vi "pH电极校准.vi"() -> ()   [LabVIEW 2016, in "斯坦道多参数.lvlib"]
uses:
  <vilib>/Utility/miscctls.llb/LVPointTypeDef.ctl
  <vilib>/Analysis/NI_AALBase.lvlib
panel:
  out "滤波设定":dbl
  in  "刷新按钮":bool
  out "第三点信号值":dbl
  out "第二点信号值":dbl
  out "第一点信号值":dbl
  out "温度":dbl format="%#.2f"
  out "通讯状态":string
  out "电极状态标志":u16(ring) items=["OK", "第一点校正通过", "第二点校正通过", "校正失败,电极零点超出范围", "校正失败,电极斜率超出范围", "第三点校正通过"]
  in  "三点标液3":u16(ring)=6 caption="标液3" items=["TECH4.00", "TECH7.00", "TECH10.00", "NIST1.68", "NIST4.01", "NIST6.86", "NIST9.18", "NIST12.68"]
  in  "三点标液2":u16(ring)=5 caption="标液2" items=["TECH4.00", "TECH7.00", "TECH10.00", "NIST1.68", "NIST4.01", "NIST6.86", "NIST9.18", "NIST12.68"]
  in  "三点标液1":u16(ring)=4 caption="标液1" items=["TECH4.00", "TECH7.00", "TECH10.00", "NIST1.68", "NIST4.01", "NIST6.86", "NIST9.18", "NIST12.68"]
  out "第三点校准值":dbl
  in  "校准停止":bool
  in  "校准启动":bool
  out "第二点校准值":dbl
  out "第一点校准值":dbl
  out "提示":string
  in  "校准模式":u16(ring) items=["两点校准", "单点校准", "三点校准"]
  out "最小值":sgl format="%#.2f"
  out "最大值":sgl format="%#.2f"
  out "变异系数":dbl format="%#.6f"
  out "standard deviation":dbl caption="标准差" format="%#.2f"
  out "mean":dbl caption="均值" format="%#.2f"
  out "波形图表":sgl(graph) caption="历史曲线"
  out "当前检测值":dbl caption="测量值" format="%#.2f"
  out "标液2":dbl
  out "标液1":dbl
  out "当前信号值":dbl caption="信号值" format="%#.2f"
  out "偏移值补偿":dbl caption="pH偏移修正值" format="%#.2f"
  out "电极斜率":dbl format="%#.6f"
  out "电极零点":dbl format="%#.6f"
  # "酸碱度电极设定"
  # "℃"
  # "mV"
  # "mV"
  # "%"
  # "请选择校准模式:"
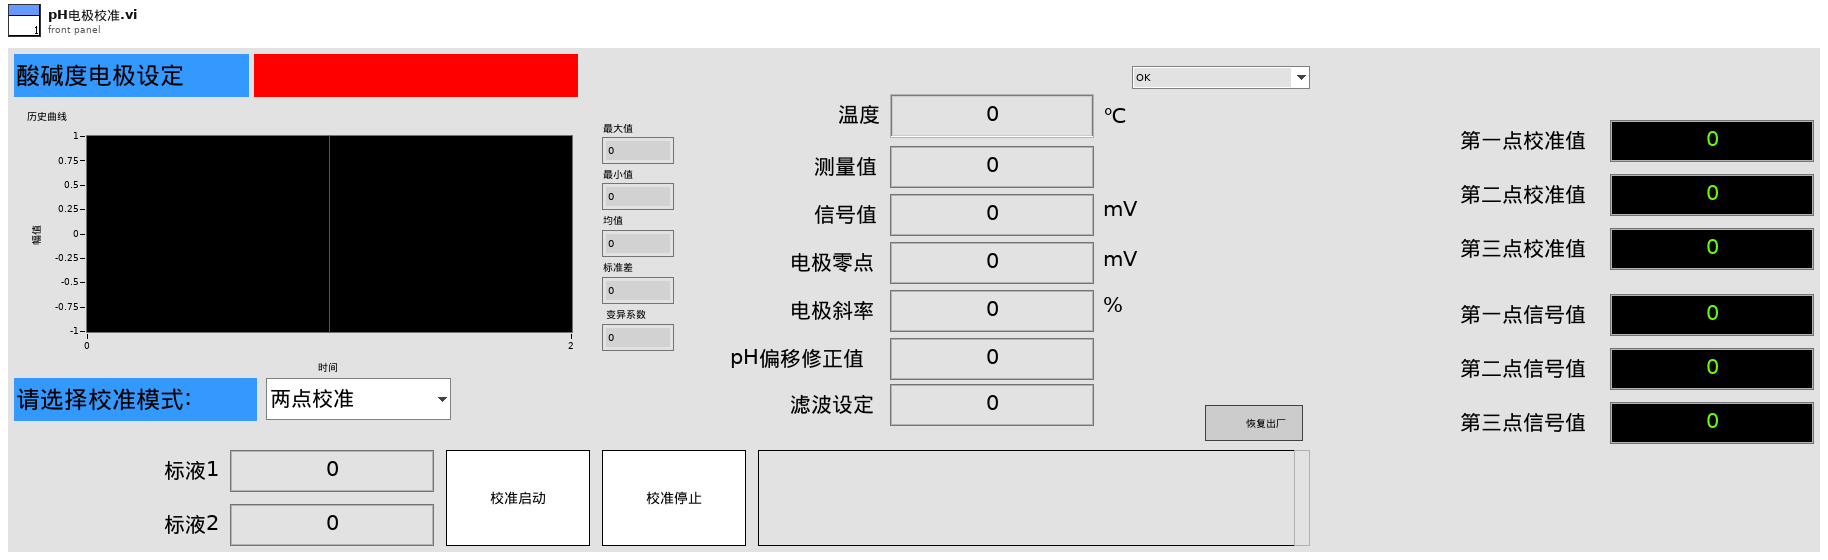
[diagram p1: front panel]
types:
  T1 = enum16{"pH", "DO", "Cond", "Turb", "ORP", "叶绿素a", "藻密度"}
  T2 = typedef "LVPointTypeDef.ctl" = cluster{"Horizontal":i16, "Vertical":i16}
  T3 = cluster{"电极状态标志":u16, "电极型号标志":u16, "酸碱度测量值":sgl, "温度测量值":sgl, "酸碱度信号值":sgl, "温度信号值":sgl, "酸碱度偏移修正值":sgl, "温度偏移修正值":sgl, "手动温度补偿值":sgl, "酸碱度电极零点":sgl, "酸碱度电极斜率":sgl, "第1点标准值记录":sgl, "第1点信号值记录":sgl, "第1点温度值记录":sgl, "第2点标准值记录":sgl, "第2点信号值记录":sgl, "第2点温度值记录":sgl, "命令滤波设定":u16, "温度模式":enum16{"ATC", "MTC"}, "生产批次":u16, "电极序号":u16, "串口地址":u16, "串口波特率":enum16{"9600", "19200", "115200"}, "串口校验位":enum16{"NONE", "ODD", "EVEN"}, "串口停止位":enum16{"1bit", "2bit"}, "第一点标准值":sgl, "第二点标准值":sgl}
  T4 = enum8{"Enabled", "Disabled", "Disabled and Grayed Out"}
  T5 = cluster{"测量量程":dbl, "测量精度":dbl, "测量间隔":dbl, "消解温度":dbl, "消解时长":dbl, "空白校准时间":timestamp, "曲线截距":dbl, "曲线斜率":dbl, "测量检出限":dbl, "测量信号值":dbl, "线性相关系数":dbl, "二次多项式系数":dbl, "标样校准时间":timestamp, "稀释倍数":dbl, "三项式系数":dbl, "空白标定系数":dbl, "量程系数":dbl, "F0/ORPA":dbl, "F1/ORPB":dbl, "F2/ORPK":dbl, "F3":dbl, "F4":dbl, "F5":dbl, "F6":dbl, "F7":dbl, "X0/滴定数":dbl, "量程":dbl}
  T6 = cluster{"ph":bool, "DO":bool, "Cond":bool, "Turb":bool, "叶绿素a":bool, "藻密度":bool, "ORP":bool}
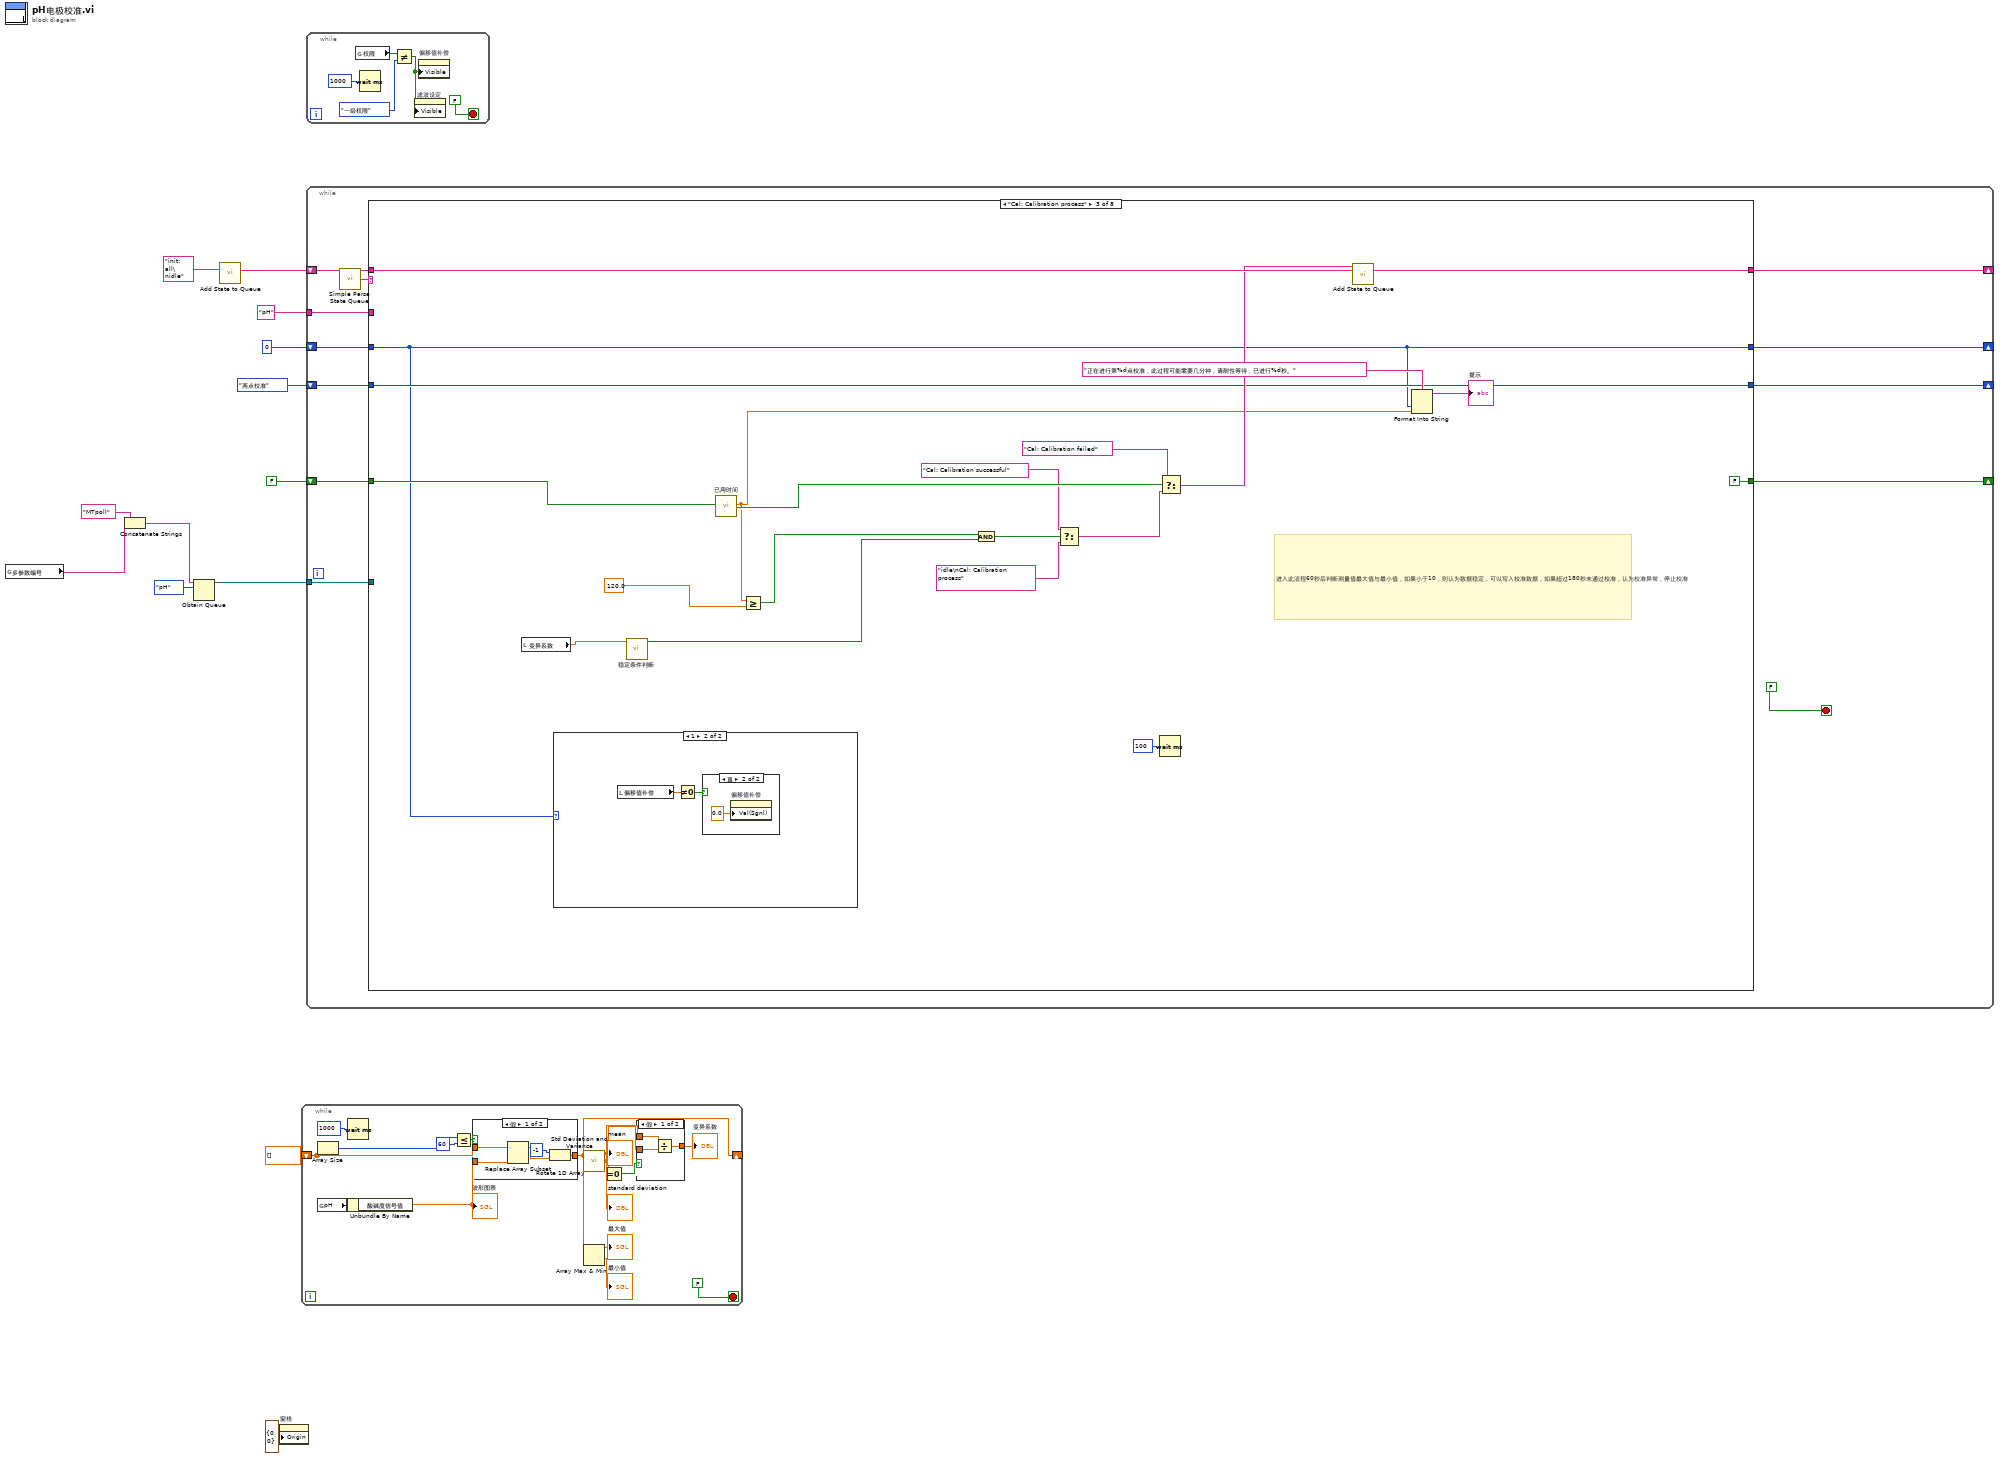
[diagram p0: block diagram]
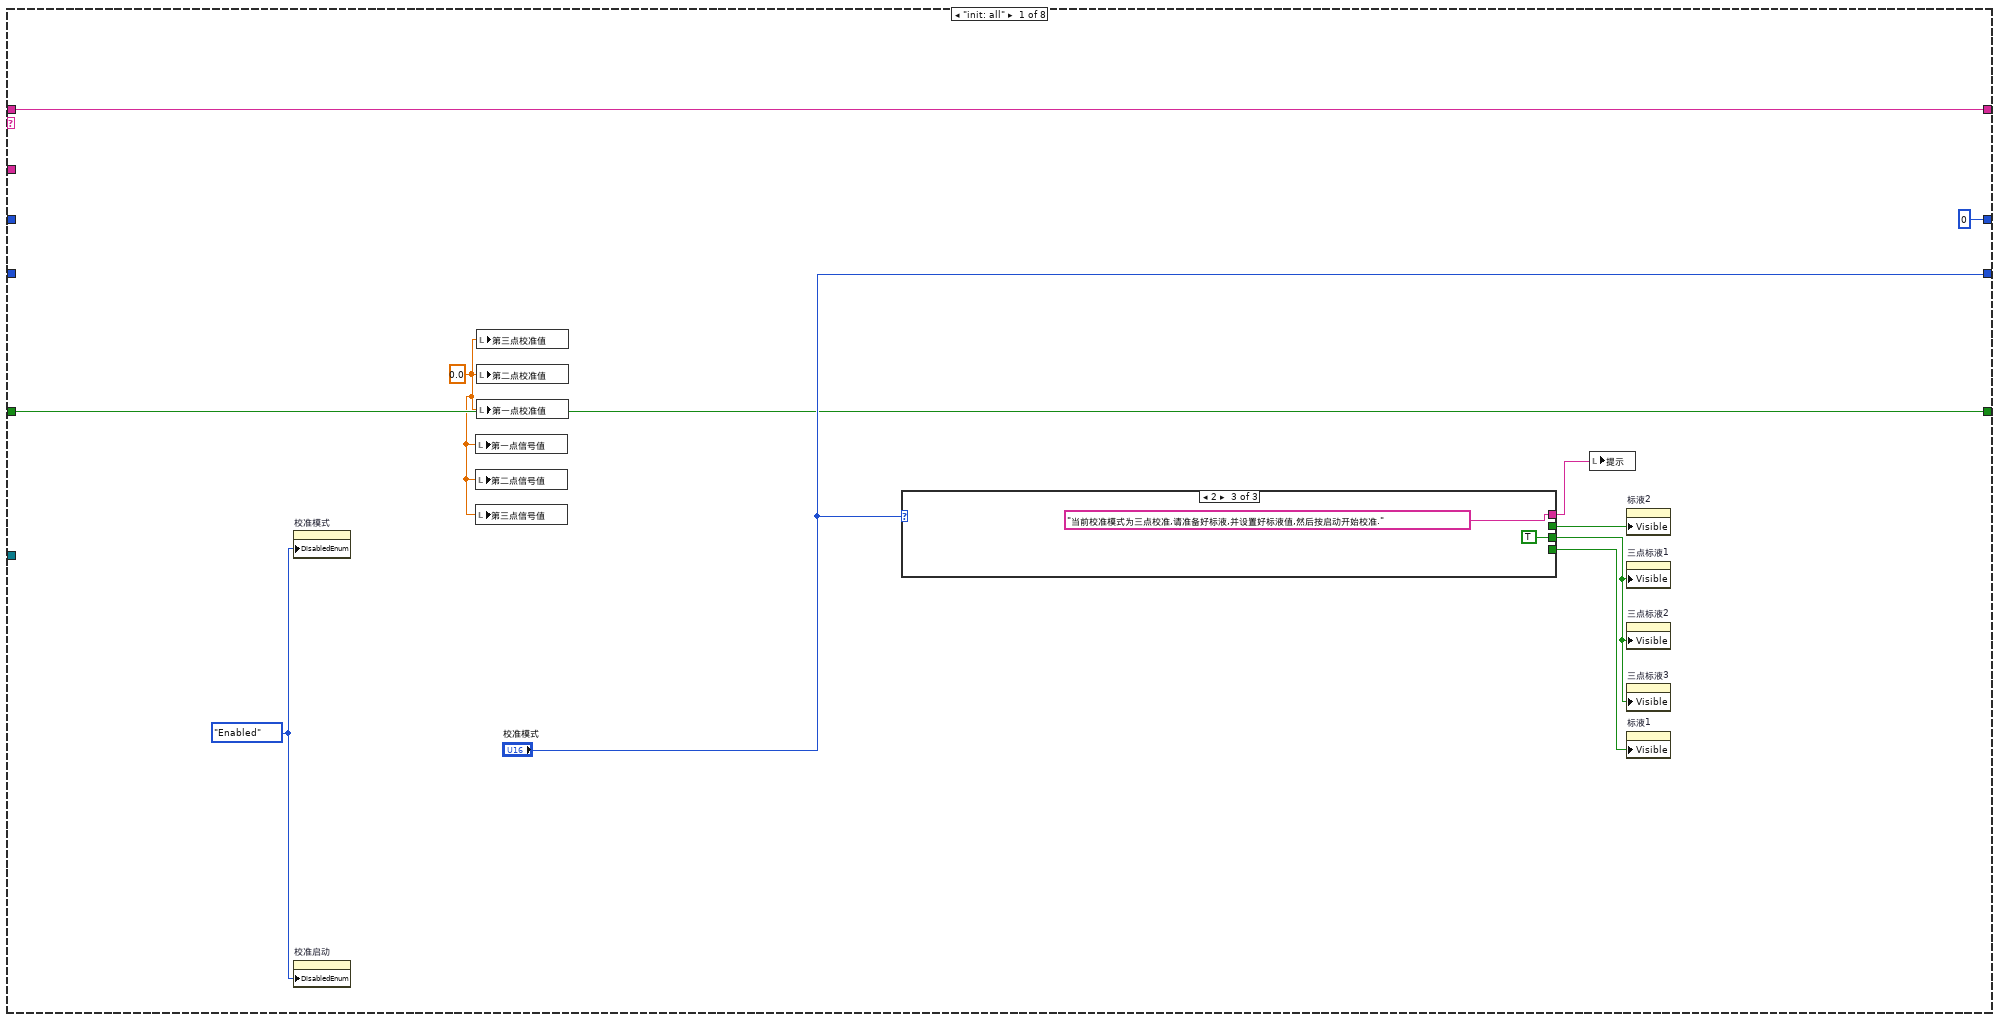
[diagram p2: hidden frame]
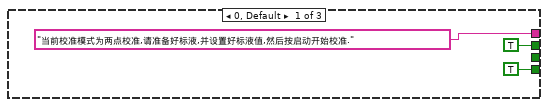
[diagram p3: hidden frame]
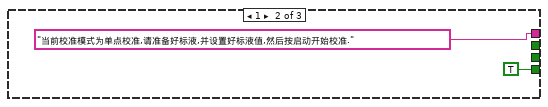
[diagram p4: hidden frame]
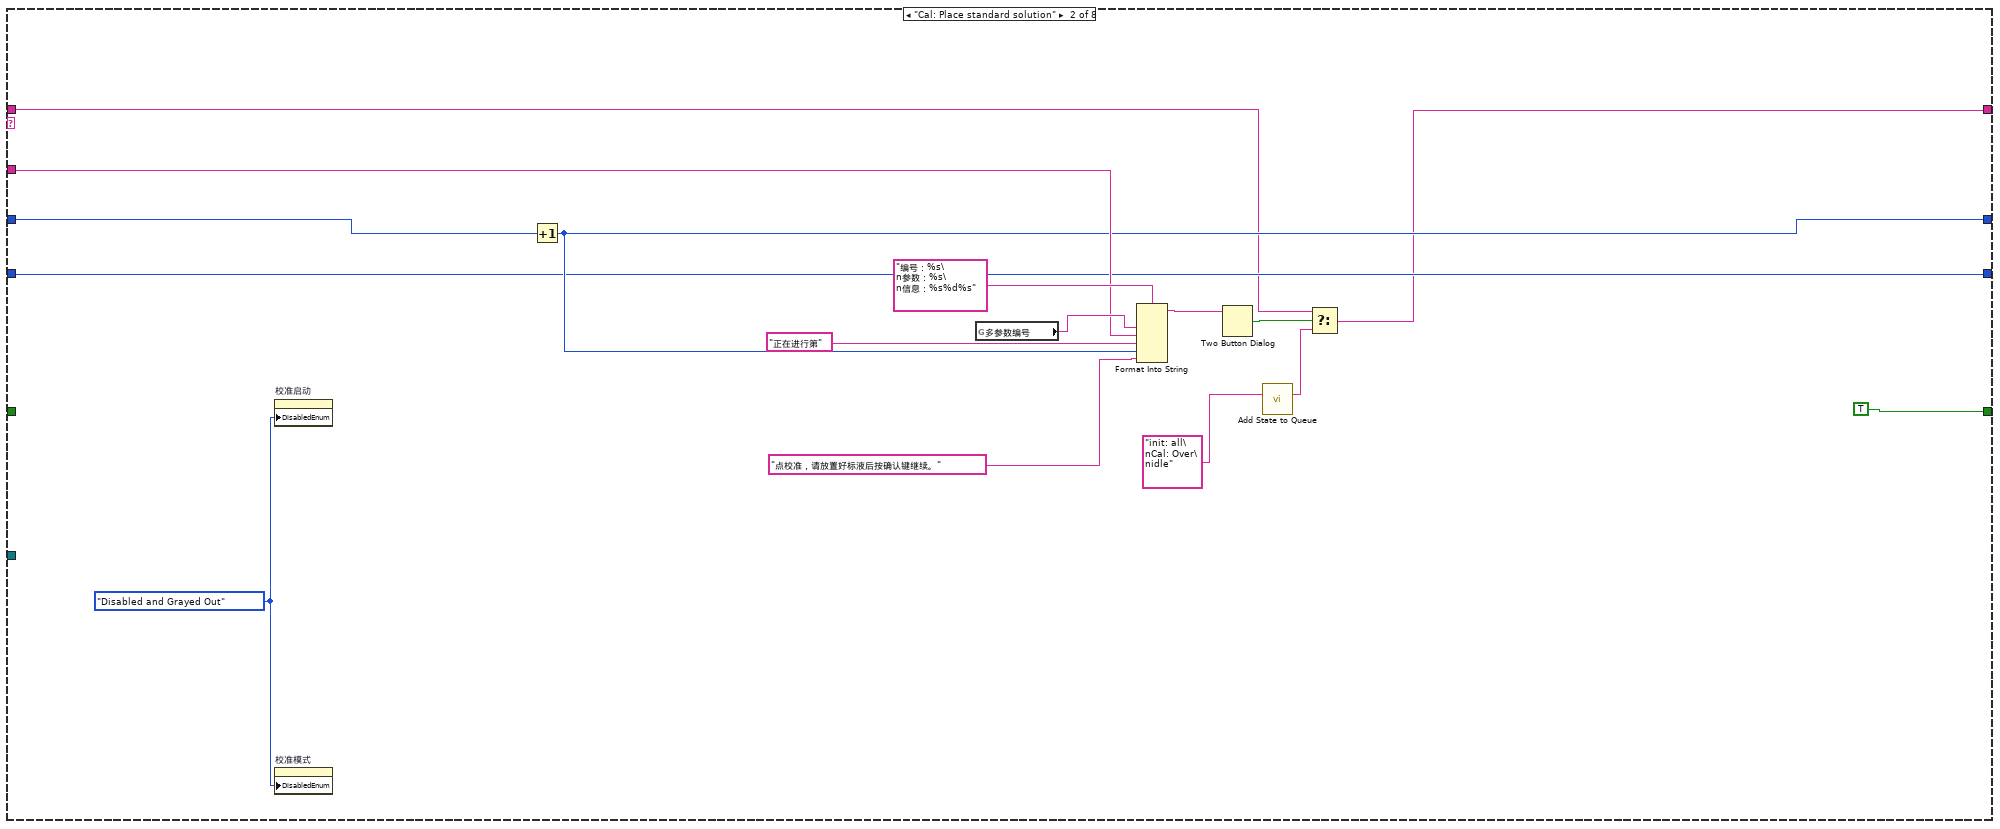
[diagram p5: hidden frame]
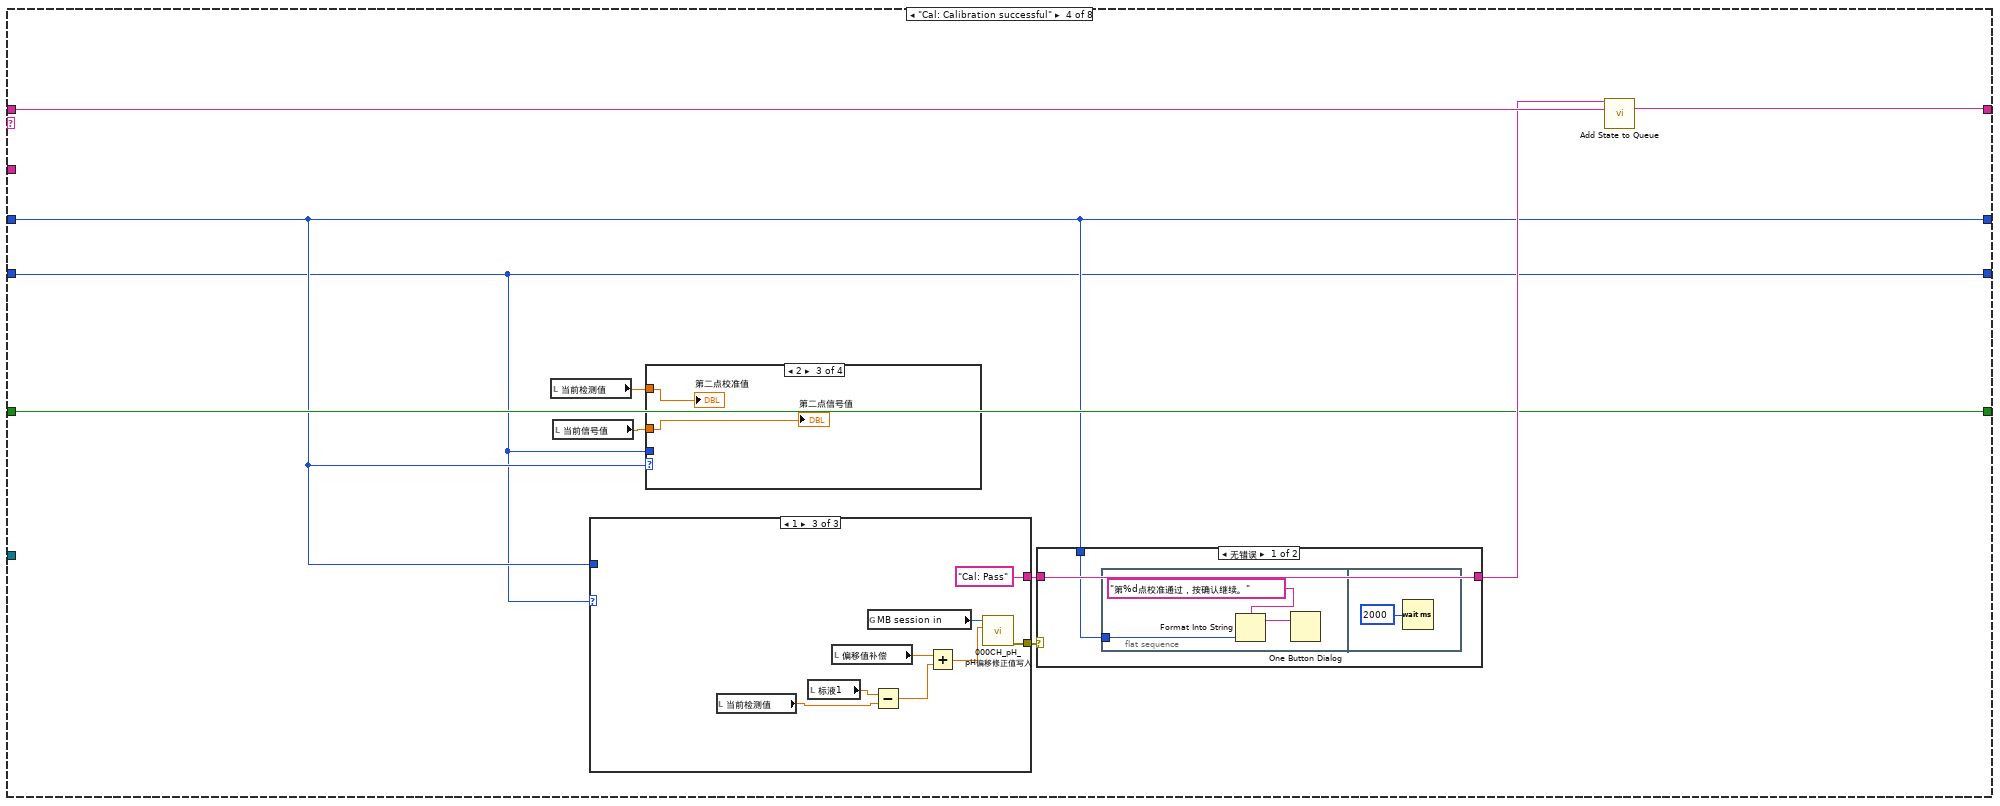
[diagram p8: hidden frame]
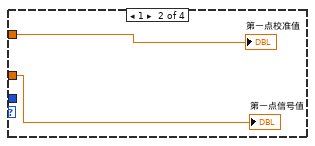
[diagram p10: hidden frame]
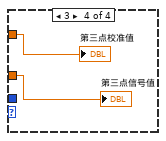
[diagram p11: hidden frame]
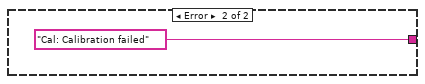
[diagram p12: hidden frame]
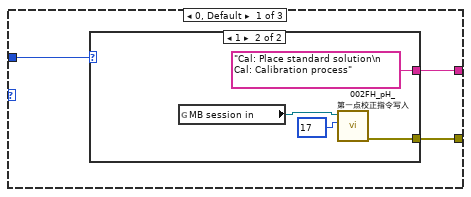
[diagram p13: hidden frame]
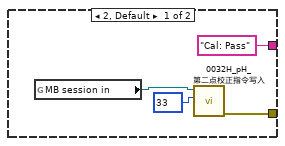
[diagram p14: hidden frame]
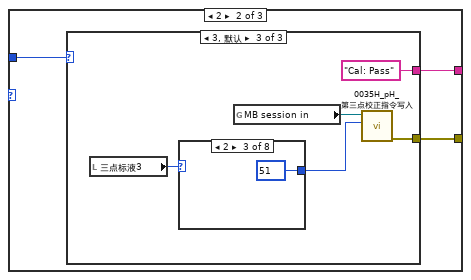
[diagram p15: hidden frame]
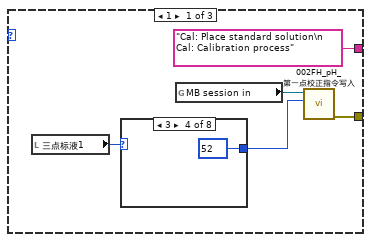
[diagram p16: hidden frame]
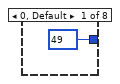
[diagram p17: hidden frame]
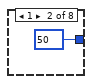
[diagram p18: hidden frame]
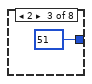
[diagram p19: hidden frame]
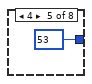
[diagram p20: hidden frame]
diagram:
  n1 = global read "多参数全局变量.vi" "多参数编号"() -> (w2:string)
  n2 = Concatenate Strings("MTpoll" ("名称（未命名）"), w2) -> (w4:string)
  n3 = Obtain Queue(name (unnamed)=w4, element data type=T1."pH" ("枚举")) -> (queue out=w1:refnum<queue>)  [unwired: 3 in, 2 out]
  n4 = call "Add State to Queue.vi"("State(s) In (\"\")"="init: all\nidle" ("State(s) In (\"\")")) -> ("States Out"=w10:string)  [unwired: 14 in]
  n5 = property on="窗格" class="Pane"("Origin"=T2 {"Horizontal"=0, "Vertical"=0} ("原点")) -> ()  [unwired: 2 in, 2 out]
  n6 = while {
    shift-right: [w20] -> _
    shift-left: sgl[] [] -> [w24]
    stop <- FALSE stop-if-true
    n7 = Array Size(array=w24) -> (size(s)=w26:i32)
    n8 = global read "国弘过程全局变量.vi" "pH"() -> (w21:T3)
    n9 = Wait (ms)(milliseconds to wait=u32 1000 ("等待时间（毫秒）")) -> ()  [unwired: 1 out]
    n10 = Unbundle By Name(w21) -> ("酸碱度信号值"=w14:sgl)
    "波形图表" <- w14
    n11 = Less Or Equal?(x=w26, y=60) -> (x <= y?=w25:bool)
    n12 = case shown="假" w25 {
      tunnel: w24 -> [w36 w39]
      tunnel: w14 -> [w34 w38]
      tunnel: [w32 w37] -> w20
      frame False {
        n13 = Replace Array Subset(array=w36, new element=w34) -> (w35:sgl[])  [unwired: 1 in]
        n14 = Rotate 1D Array(1:w35, 2:-1 ("n")) -> (0:w32:sgl[])
      }
      frame True {
        n15 = Insert Into Array(array=w39, new element=w38) -> (w37:sgl[])  [unwired: 1 in]
      }
    }
    n16 = call <vilib>:"Std Deviation and Variance.vi"("X"=w20) -> ("mean"=w16:dbl, "standard deviation"=w15:dbl)  [unwired: 1 in, 1 out]
    "mean" <- w16
    "standard deviation" <- w15
    n17 = Array Max & Min(array=w20) -> (max value=→"最大值":sgl, min value=→"最小值":sgl)  [unwired: 2 out]
    n18 = Equal To 0?(x=w16) -> (x = 0?=w23:bool)
    n19 = case shown="假" w23 {
      tunnel: w15 -> [w31 _]
      tunnel: [w30 _] -> w17
      tunnel: w16 -> [w29 _]
      frame False {
        n20 = Divide(x=w31, y=w29) -> (x/y=w30:dbl)
      }
      frame True {
      }
    }
    "变异系数" <- w17
  }
  n21 = while {
    shift-right: [w48] -> _
    shift-left: w10 -> [w52]
    shift-right: [w45] -> _
    shift-left: 0 -> [w47]
    tunnel: "pH" ("State(s) In (\"\")") -> [w46]
    shift-right: [w43] -> _
    shift-left: enum16{"两点校准", "单点校准", "三点校准"}."两点校准" ("校准模式") -> [w44]
    shift-right: [w41] -> _
    shift-left: FALSE -> [w42]
    tunnel: w1 -> [w40]
    stop <- FALSE stop-if-true
    n22 = call "Simple Parse State Queue.vi"("State Queue"=w52) -> ("Remain States"=w49:string, "Next State"=w50:string)  [unwired: 13 in]
    n23 = case shown="\"Cal: Calibration process\"" w50 {
      tunnel: w49 -> [w62 w72 w105 w117 _ _ w265 w276]
      tunnel: [w62 w71 w104 w116 w201 w211 w265 w275] -> w48
      tunnel: w47 -> [_ w81 w89 w111 w204 w220 w264 w273]
      tunnel: w46 -> [_ w82 _ _ w195 w216 _ _]
      tunnel: [0 w79 w89 w111 w204 w220 w264 w274] -> w45
      tunnel: w44 -> [_ w78 w90 w110 w203 w212 w263 w272]
      tunnel: ["校准模式" w78 w90 w110 w203 w212 w263 w272] -> w43
      tunnel: w42 -> [w55 _ w92 w112 w202 w215 w262 w270]
      tunnel: [w55 TRUE FALSE w112 w202 w215 w262 w270] -> w41
      tunnel: w40 -> [_ _ _ _ _ _ _ w269]
      frame "init: all" {
        w54 = T4."Enabled" ("禁用")
        w53 = 0.0 ("第一点校准值")
        n24 = property on="校准模式" class="Ring (严格)"("DisabledEnum"=w54) -> ()  [unwired: 2 in, 2 out]
        n25 = property on="校准启动" class="Bool"("DisabledEnum"=w54) -> ()  [unwired: 2 in, 2 out]
        n26 = local write "第一点信号值"(w53) -> ()
        n27 = local write "第二点信号值"(w53) -> ()
        n28 = local write "第三点信号值"(w53) -> ()
        n29 = local write "第三点校准值"(w53) -> ()
        n30 = local write "第二点校准值"(w53) -> ()
        n31 = local write "第一点校准值"(w53) -> ()
        n32 = case shown="2" "校准模式" {
          tunnel: ["当前校准模式为两点校准,请准备好标液,并设置好标液值,然后按启动开始校准." ("提示") "当前校准模式为单点校准,请准备好标液,并设置好标液值,然后按启动开始校准." ("提示") "当前校准模式为三点校准,请准备好标液,并设置好标液值,然后按启动开始校准." ("提示")] -> w57
          tunnel: [TRUE ("可见") _ _] -> w61
          tunnel: [TRUE ("可见") TRUE ("可见") _] -> w59
          tunnel: [_ _ TRUE ("可见")] -> w60
          frame 0, Default {
          }
          frame 1 {
          }
          frame 2 {
          }
        }
        n33 = local write "提示"(w57) -> ()
        n34 = property on="标液2" class="DigNum (严格)"("Visible"=w61) -> ()  [unwired: 2 in, 2 out]
        n35 = property on="三点标液1" class="Ring (严格)"("Visible"=w60) -> ()  [unwired: 2 in, 2 out]
        n36 = property on="三点标液2" class="Ring (严格)"("Visible"=w60) -> ()  [unwired: 2 in, 2 out]
        n37 = property on="三点标液3" class="Ring (严格)"("Visible"=w60) -> ()  [unwired: 2 in, 2 out]
        n38 = property on="标液1" class="DigNum (严格)"("Visible"=w59) -> ()  [unwired: 2 in, 2 out]
      }
      frame "Cal: Place standard solution" {
        w76 = T4."Disabled and Grayed Out" ("禁用")
        n39 = property on="校准启动" class="Bool"("DisabledEnum"=w76) -> ()  [unwired: 2 in, 2 out]
        n40 = property on="校准模式" class="Ring (严格)"("DisabledEnum"=w76) -> ()  [unwired: 2 in, 2 out]
        n41 = Increment(x=w81) -> (x+1=w79:i32)
        n42 = global read "多参数全局变量.vi" "多参数编号"() -> (w84:string)
        n43 = Format Into String(format string="编号：%s\n参数：%s\n信息：%s%d%s" ("格式字符串"), w84, w82, "正在进行第" ("消息"), w79, "点校准，请放置好标液后按确认键继续。" ("消息")) -> (resulting string=w75:string)  [unwired: 2 in, 1 out]
        n44 = Two Button Dialog(message=w75) -> (T button?=w74:bool)  [unwired: 2 in]
        n45 = call "Add State to Queue.vi"("State(s) In (\"\")"="init: all\nCal: Over\nidle" ("State(s) In (\"\")")) -> ("States Out"=w73:string)  [unwired: 14 in]
        n46 = Select(t=w72, s=w74, f=w73) -> (s? t:f=w71:string)
      }
      frame "Cal: Calibration process" {
        # "进入此流程60秒后判断测量值最大值与最小值，如果小于10，则认为数据稳定，可以写入校准数据，如果超过180秒未通过校准，认为校准异常，停止校准"
        n47 = local read "变异系数"() -> (w87:dbl)
        n48 = case shown="1" w89 {
          frame 0, Default {
          }
          frame 1 {
            n49 = local read "偏移值补偿"() -> (w107:dbl)
            n50 = Not Equal To 0?(x=w107) -> (x != 0?=w108:bool)
            n51 = case shown="真" w108 {
              frame False {
              }
              frame True {
                n52 = property on="偏移值补偿" class="DigNum (严格)"("Val(Sgnl)"=0.0 ("值(信号)")) -> ()  [unwired: 2 in, 2 out]
              }
            }
          }
        }
        n53 = call "稳定条件判断.vi"("变异系数"=w87) -> ("布尔"=w86:bool)  [unwired: 10 in]
        n54 = call "已用时间"("Reset"=w92) -> ("Elapsed Time (s)"=w88:dbl, "Time has Elapsed"=w106:bool)  [unwired: 11 in, 6 out]
        n55 = Greater Or Equal?(x=w88, y=120.0) -> (x >= y?=w101:bool)
        n56 = And(x=w101, y=w86) -> (x .and. y?=w98:bool)
        n57 = Select(t="Cal: Calibration successful" ("State(s) In (\"\")"), s=w98, f="idle\nCal: Calibration process" ("State(s) In (\"\")")) -> (s? t:f=w97:string)
        n58 = Wait (ms)(milliseconds to wait=u32 100 ("等待时间（毫秒）")) -> ()  [unwired: 1 out]
        n59 = Select(t="Cal: Calibration failed" ("State(s) In (\"\")"), s=w106, f=w97) -> (s? t:f=w96:string)
        n60 = call "Add State to Queue.vi"("State(s) In Front (\"\")"=w96, "State(s) In (\"\")"=w105) -> ("States Out"=w104:string)  [unwired: 13 in]
        n61 = Format Into String(format string="正在进行第%d点校准，此过程可能需要几分钟，请耐性等待，已进行%d秒。" ("格式字符串"), w89, w88) -> (resulting string=→"提示":string)  [unwired: 2 in, 1 out]
      }
      frame "Cal: Calibration successful" {
        n62 = local read "当前检测值"() -> (w113:dbl)
        n63 = local read "当前信号值"() -> (w114:dbl)
        n64 = case shown="1" w110 {
          tunnel: [w135 w146 w188] -> w119
          tunnel: [w134 w144 "Cal: Pass" ("State(s) In (\"\")")] -> w118
          tunnel: w111 -> [w133 w145 _]
          frame 0, Default {
            n65 = case shown="1" w133 {
              tunnel: [w136 w141] -> w135
              tunnel: ["Cal: Pass" ("State(s) In (\"\")") "Cal: Place standard solution\n Cal: Calibration process" ("State(s) In (\"\")")] -> w134
              frame 2, Default {
                n66 = global read "多参数全局变量.vi" "MB session in"() -> (w138:refnum<class "MB_Master.lvclass">)
                n67 = call "0032H_pH_第二点校正指令写入.vi"("数值"=u16 33, "MB session in"=w138) -> ("error out"=w136:errorcluster)  [unwired: 8 in, 1 out]
              }
              frame 1 {
                n68 = global read "多参数全局变量.vi" "MB session in"() -> (w143:refnum<class "MB_Master.lvclass">)
                n69 = call "002FH_pH_第一点校正指令写入.vi"("数值"=u16 17, "MB session in"=w143) -> ("error out"=w141:errorcluster)  [unwired: 8 in, 1 out]
              }
            }
          }
          frame 2 {
            n70 = case shown="3, 默认" w145 {
              tunnel: [w148 w161 w174] -> w146
              tunnel: ["Cal: Place standard solution\n Cal: Calibration process" ("State(s) In (\"\")") "Cal: Place standard solution\n Cal: Calibration process" ("State(s) In (\"\")") "Cal: Pass" ("State(s) In (\"\")")] -> w144
              frame 1 {
                n71 = local read "三点标液1"() -> (w150:u16)
                n72 = case shown="3" w150 {
                  tunnel: [u16 49 ("数值") u16 50 ("数值") u16 51 ("数值") u16 52 ("数值") u16 53 ("数值") u16 54 ("数值") u16 55 ("数值") u16 56 ("数值")] -> w149
                  frame 0, Default {
                  }
                  frame 1 {
                  }
                  frame 2 {
                  }
                  frame 3 {
                  }
                  frame 4 {
                  }
                  frame 5 {
                  }
                  frame 6 {
                  }
                  frame 7 {
                  }
                }
                n73 = global read "多参数全局变量.vi" "MB session in"() -> (w151:refnum<class "MB_Master.lvclass">)
                n74 = call "002FH_pH_第一点校正指令写入.vi"("数值"=w149, "MB session in"=w151) -> ("error out"=w148:errorcluster)  [unwired: 8 in, 1 out]
              }
              frame 2 {
                n75 = local read "三点标液2"() -> (w163:u16)
                n76 = case shown="7" w163 {
                  tunnel: [u16 49 ("数值") u16 50 ("数值") u16 51 ("数值") u16 52 ("数值") u16 53 ("数值") u16 54 ("数值") u16 55 ("数值") u16 56 ("数值")] -> w162
                  frame 0, Default {
                  }
                  frame 1 {
                  }
                  frame 2 {
                  }
                  frame 3 {
                  }
                  frame 4 {
                  }
                  frame 5 {
                  }
                  frame 6 {
                  }
                  frame 7 {
                  }
                }
                n77 = global read "多参数全局变量.vi" "MB session in"() -> (w164:refnum<class "MB_Master.lvclass">)
                n78 = call "0032H_pH_第二点校正指令写入.vi"("数值"=w162, "MB session in"=w164) -> ("error out"=w161:errorcluster)  [unwired: 8 in, 1 out]
              }
              frame 3, Default {
                n79 = local read "三点标液3"() -> (w176:u16)
                n80 = case shown="2" w176 {
                  tunnel: [u16 49 ("数值") u16 50 ("数值") u16 51 ("数值") u16 52 ("数值") u16 53 ("数值") u16 54 ("数值") u16 55 ("数值") u16 56 ("数值")] -> w175
                  frame 0, Default {
                  }
                  frame 1 {
                  }
                  frame 2 {
                  }
                  frame 3 {
                  }
                  frame 4 {
                  }
                  frame 5 {
                  }
                  frame 6 {
                  }
                  frame 7 {
                  }
                }
                n81 = global read "多参数全局变量.vi" "MB session in"() -> (w177:refnum<class "MB_Master.lvclass">)
                n82 = call "0035H_pH_第三点校正指令写入.vi"("数值"=w175, "MB session in"=w177) -> ("error out"=w174:errorcluster)  [unwired: 8 in, 1 out]
              }
            }
          }
          frame 1 {
            n83 = local read "当前检测值"() -> (w186:dbl)
            n84 = local read "标液1"() -> (w193:dbl)
            n85 = local read "偏移值补偿"() -> (w189:dbl)
            n86 = global read "多参数全局变量.vi" "MB session in"() -> (w192:refnum<class "MB_Master.lvclass">)
            n87 = Subtract(x=w193, y=w186) -> (x-y=w191:dbl)
            n88 = Add(x=w189, y=w191) -> (x+y=w190:dbl)
            n89 = call "000CH_pH_pH偏移修正值写入.vi"("数值"=w190, "MB session in"=w192) -> ("error out"=w188:errorcluster)  [unwired: 8 in, 1 out]
          }
        }
        n90 = case shown="2" w111 {
          tunnel: w114 -> [_ w121 w122 w124]
          tunnel: w113 -> [_ w120 w123 w125]
          tunnel: w110 -> [_ _ _ _]
          frame 0, Default {
          }
          frame 1 {
            "第一点校准值" <- w120
            "第一点信号值" <- w121
          }
          frame 2 {
            "第二点校准值" <- w123
            "第二点信号值" <- w122
          }
          frame 3 {
            "第三点校准值" <- w125
            "第三点信号值" <- w124
          }
        }
        n91 = case shown="无错误" w119 {
          tunnel: w118 -> [w127 _]
          tunnel: [w127 "Cal: Calibration failed" ("State(s) In (\"\")")] -> w115
          tunnel: w111 -> [w126 _]
          frame No Error {
            n92 = flat-sequence {
              tunnel: w126 -> [w128]
              frame #0 {
                n93 = Format Into String(format string="第%d点校准通过，按确认继续。" ("格式字符串"), w128) -> (resulting string=w130:string)  [unwired: 2 in, 1 out]
                n94 = One Button Dialog(message=w130) -> ()  [unwired: 1 in, 1 out]
              }
              frame #1 {
                n95 = Wait (ms)(milliseconds to wait=u32 2000 ("等待时间（毫秒）")) -> ()  [unwired: 1 out]
              }
            }
          }
          frame Error {
          }
        }
        n96 = call "Add State to Queue.vi"("State(s) In Front (\"\")"=w115, "State(s) In (\"\")"=w117) -> ("States Out"=w116:string)  [unwired: 13 in]
      }
      frame "Cal: Calibration failed" {
        n97 = global read "多参数全局变量.vi" "多参数编号"() -> (w198:string)
        n98 = call "Add State to Queue.vi"("State(s) In (\"\")"="init: all\nCal: Over\nidle" ("State(s) In (\"\")")) -> ("States Out"=w201:string)  [unwired: 14 in]
        n99 = Format Into String(format string="编号：%s\n参数：%s\n信息：%s" ("格式字符串"), w198, w195, "校准失败！" ("消息")) -> (resulting string=w197:string)  [unwired: 2 in, 1 out]
        n100 = One Button Dialog(message=w197) -> ()  [unwired: 1 in, 1 out]
        n101 = call "校准日志.vi"("table"="校准记录", "日志信息"=w197) -> ()  [unwired: 9 in, 1 out]
      }
      frame "Cal: Pass" {
        n102 = flat-sequence {
          tunnel: [w225] -> w213
          tunnel: w212 -> [w224]
          tunnel: [w223] -> w210
          tunnel: [w222] -> w209
          frame #0 {
            n103 = Wait (ms)(milliseconds to wait=u32 3000 ("等待时间（毫秒）")) -> ()  [unwired: 1 out]
          }
          frame #1 {
            n104 = global read "国弘过程全局变量.vi" "pH"() -> (w226:T3)
            n105 = Unbundle By Name(w226) -> ("电极状态标志"=w227:u16, "酸碱度电极零点"=w223:sgl, "酸碱度电极斜率"=w222:sgl)
            n106 = case shown="0, 默认" w224 {
              tunnel: [w229 w244 w261] -> w225
              tunnel: w227 -> [w228 w243 _]
              frame 0, Default {
                n107 = case shown="2" w228 {
                  selector: w228 -> [_ _ w240]
                  tunnel: ["校准异常，校准未完成。" ("格式字符串") w238 w239] -> w229
                  frame 0, Default {
                  }
                  frame 2 {
                    n108 = local read "第一点校准值"() -> (w236:dbl)
                    n109 = local read "第一点信号值"() -> (w237:dbl)
                    n110 = local read "第二点校准值"() -> (w233:dbl)
                    n111 = local read "第二点信号值"() -> (w232:dbl)
                    n112 = local read "标液1"() -> (w234:dbl)
                    n113 = local read "标液2"() -> (w231:dbl)
                    n114 = Format Into String(format string="校准结果：\n第一点校准值=%#.2f，第一点信号值=%#.2f mV，第一点标准值=%#.2f；\n第二点校准值=%#.2f，第二点信号值=%#.2f mV，第二点标准值=%#.2f。" ("提示"), w236, w237, w234, w233, w232, w231) -> (resulting string=w238:string)  [unwired: 2 in, 1 out]
                  }
                  frame 3, 4 {
                    n115 = case shown="4" w240 {
                      tunnel: ["校正失败，电极零点超出范围" "校正失败，电极斜率超出范围"] -> w239
                      frame 3, Default {
                      }
                      frame 4 {
                      }
                    }
                  }
                }
              }
              frame 2 {
                n116 = case shown="5" w243 {
                  tunnel: ["校准异常，校准未完成。" ("格式字符串") w256] -> w244
                  frame 0, Default {
                  }
                  frame 5 {
                    n117 = local read "第一点校准值"() -> (w255:dbl)
                    n118 = local read "第一点信号值"() -> (w253:dbl)
                    n119 = local read "第二点校准值"() -> (w251:dbl)
                    n120 = local read "第二点信号值"() -> (w250:dbl)
                    n121 = local read "第三点校准值"() -> (w248:dbl)
                    n122 = local read "第三点信号值"() -> (w247:dbl)
                    n123 = property on="三点标液1" class="Ring (严格)"() -> ("RingText.Text"=w252:string)  [unwired: 2 in, 2 out]
                    n124 = property on="三点标液2" class="Ring (严格)"() -> ("RingText.Text"=w249:string)  [unwired: 2 in, 2 out]
                    n125 = property on="三点标液3" class="Ring (严格)"() -> ("RingText.Text"=w246:string)  [unwired: 2 in, 2 out]
                    n126 = Format Into String(format string="校准结果：\n第一点校准值=%#.2f，第一点信号值=%#.2f mV，第一点标准值=%s；\n第二点校准值=%#.2f，第二点信号值=%#.2f mV，第二点标准值=%s；\n第三点校准值=%#.2f，第三点信号值=%#.2f mV，第三点标准值=%s。" ("提示"), w255, w253, w252, w251, w250, w249, w248, w247, w246) -> (resulting string=w256:string)  [unwired: 2 in, 1 out]
                  }
                }
              }
              frame 1 {
                n127 = local read "第一点校准值"() -> (w260:dbl)
                n128 = local read "第一点信号值"() -> (w258:dbl)
                n129 = local read "标液1"() -> (w257:dbl)
                n130 = Format Into String(format string="校准结果：\n校准值=%#.2f，信号值=%#.2f，标准值=%#.2f。" ("提示"), w260, w258, w257) -> (resulting string=w261:string)  [unwired: 2 in, 1 out]
              }
            }
          }
        }
        n131 = Get Date/Time In Seconds() -> (seconds since 1Jan1904=w205:timestamp)
        n132 = global read "断电保存变量.vi" "PH参数"() -> (w207:T5)
        n133 = Bundle By Name(cluster=w207, "空白校准时间"=w205, "标样校准时间"=w205) -> (w206:T5)
        n134 = global write "断电保存变量.vi" "PH参数"(w206) -> ()
        n135 = call "Add State to Queue.vi"("State(s) In (\"\")"="init: all\nCal: Over\nidle" ("State(s) In (\"\")")) -> ("States Out"=w211:string)  [unwired: 14 in]
        n136 = global read "多参数全局变量.vi" "多参数编号"() -> (w217:string)
        n137 = Format Into String(format string="编号：%s\n参数：%s\n信息：%s\n电极零点=%#.2f，电极斜率=%#.2f%%。" ("格式字符串"), w217, w216, w213, w210, w209) -> (resulting string=w214:string)  [unwired: 2 in, 1 out]
        n138 = One Button Dialog(message=w214) -> ()  [unwired: 1 in, 1 out]
        n139 = call "校准日志.vi"("table"="校准记录", "日志信息"=w214) -> ()  [unwired: 9 in, 1 out]
      }
      frame "Cal: Over" {
        n140 = global read "多参数全局变量.vi" "校准运行状态"() -> (w267:T6)
        n141 = Bundle By Name(cluster=w267, "ph"=FALSE) -> (w268:T6)
        n142 = global write "多参数全局变量.vi" "校准运行状态"(w268) -> ()
      }
      frame "idle", Default {
        n143 = event shown="[0] 超时" {
          selector: _ -> [_ _ _ _ _ _ _ _ _ _ _ _ _]
          dyn-events: _ -> [_ _ _ _ _ _ _ _ _ _ _ _ _]
          timeout: 10 -> [_ _ _ _ _ _ _ _ _ _ _ _ _]
          tunnel: [_ _ _ _ _ _ w361 w371 w380 w389 _ _ _] -> _
          tunnel: w276 -> [w294 w298 w299 w321 w335 w356 w368 w372 w381 w393 w398 w409 _]
          tunnel: [w293 w297 w300 w322 w336 w357 w367 w373 w382 w394 w397 w408 w411] -> w275
          tunnel: [w292 w295 w301 w323 w337 w358 w366 w374 w383 w395 w396 w406 w412] -> w274
          tunnel: w273 -> [w292 w295 w301 w323 w337 w358 w366 w374 w383 w395 w396 w406 w412]
          tunnel: w269 -> [_ _ _ _ _ _ w363 w370 w379 w388 _ _ _]
          event Timeout {
            n144 = event-data() -> ()  [unwired: 1 in, 3 out]
            n145 = global read "国弘过程全局变量.vi" "pH"() -> (w291:T3)
            n146 = Unbundle By Name(w291) -> ("电极状态标志"=→"电极状态标志":u16, "酸碱度电极零点"=→"电极零点":sgl, "酸碱度电极斜率"=→"电极斜率":sgl, "酸碱度偏移修正值"=→"偏移值补偿":sgl, "酸碱度信号值"=→"当前信号值":sgl, "第一点标准值"=→"标液1":sgl, "第二点标准值"=→"标液2":sgl, "酸碱度测量值"=→"当前检测值":sgl, "温度测量值"=→"温度":sgl, "命令滤波设定"=→"滤波设定":u16)  [unwired: 1 out]
            n147 = global read "多参数全局变量.vi" "ph通讯状态"() -> (w280:bool)
            n148 = property on="通讯状态" class="Str"("Blinking"=TRUE ("闪烁"), "Text.BG Color"=u32 16711680, "Visible"=w280) -> ()  [unwired: 2 in, 2 out]
            n149 = call "Add State to Queue.vi"("State(s) In (\"\")"=w294) -> ("States Out"=w293:string)  [unwired: 14 in]
            "通讯状态" <- "通讯异常" ("当前串口")
          }
          event "校准模式": Value Change {
            n150 = event-data() -> ()  [unwired: 1 in, 6 out]
            n151 = call "Add State to Queue.vi"("State(s) In (\"\")"=w298, "State(s) At Back (\"\")"="init: all\nidle" ("State(s) In (\"\")")) -> ("States Out"=w297:string)  [unwired: 13 in]
          }
          event "三点标液1": Value Change {
            n152 = event-data() -> ("NewVal"=w302:u16)  [unwired: 1 in, 5 out]
            n153 = case shown="1" w302 {
              frame 0, Default {
                w303 = u16 0 items=["TECH4.00", "TECH7.00", "TECH10.00", "NIST1.68", "NIST4.01", "NIST6.86", "NIST9.18", "NIST12.68"] ("标液2")
                w304 = u16 2 items=["TECH4.00", "TECH7.00", "TECH10.00", "NIST1.68", "NIST4.01", "NIST6.86", "NIST9.18", "NIST12.68"] ("标液3")
                w305 = u16 1 items=["TECH4.00", "TECH7.00", "TECH10.00", "NIST1.68", "NIST4.01", "NIST6.86", "NIST9.18", "NIST12.68"] ("标液2")
                n154 = local write "三点标液3"(w304) -> ()
                n155 = local write "三点标液2"(w305) -> ()
                n156 = local write "三点标液1"(w303) -> ()
              }
              frame 1 {
                w306 = u16 0 items=["TECH4.00", "TECH7.00", "TECH10.00", "NIST1.68", "NIST4.01", "NIST6.86", "NIST9.18", "NIST12.68"] ("标液2")
                w307 = u16 2 items=["TECH4.00", "TECH7.00", "TECH10.00", "NIST1.68", "NIST4.01", "NIST6.86", "NIST9.18", "NIST12.68"] ("标液3")
                w308 = u16 1 items=["TECH4.00", "TECH7.00", "TECH10.00", "NIST1.68", "NIST4.01", "NIST6.86", "NIST9.18", "NIST12.68"] ("标液2")
                n157 = local write "三点标液3"(w307) -> ()
                n158 = local write "三点标液2"(w308) -> ()
                n159 = local write "三点标液1"(w306) -> ()
              }
              frame 2 {
                w309 = u16 2 items=["TECH4.00", "TECH7.00", "TECH10.00", "NIST1.68", "NIST4.01", "NIST6.86", "NIST9.18", "NIST12.68"] ("标液2")
                w310 = u16 0 items=["TECH4.00", "TECH7.00", "TECH10.00", "NIST1.68", "NIST4.01", "NIST6.86", "NIST9.18", "NIST12.68"] ("标液3")
                w311 = u16 1 items=["TECH4.00", "TECH7.00", "TECH10.00", "NIST1.68", "NIST4.01", "NIST6.86", "NIST9.18", "NIST12.68"] ("标液2")
                n160 = local write "三点标液3"(w310) -> ()
                n161 = local write "三点标液2"(w311) -> ()
                n162 = local write "三点标液1"(w309) -> ()
              }
              frame 3 {
                w312 = u16 3 items=["TECH4.00", "TECH7.00", "TECH10.00", "NIST1.68", "NIST4.01", "NIST6.86", "NIST9.18", "NIST12.68"] ("标液2")
                w313 = u16 5 items=["TECH4.00", "TECH7.00", "TECH10.00", "NIST1.68", "NIST4.01", "NIST6.86", "NIST9.18", "NIST12.68"] ("标液3")
                w314 = u16 4 items=["TECH4.00", "TECH7.00", "TECH10.00", "NIST1.68", "NIST4.01", "NIST6.86", "NIST9.18", "NIST12.68"] ("标液2")
                n163 = local write "三点标液3"(w313) -> ()
                n164 = local write "三点标液2"(w314) -> ()
                n165 = local write "三点标液1"(w312) -> ()
              }
              frame 4 {
                w315 = u16 4 items=["TECH4.00", "TECH7.00", "TECH10.00", "NIST1.68", "NIST4.01", "NIST6.86", "NIST9.18", "NIST12.68"] ("标液2")
                w316 = u16 6 items=["TECH4.00", "TECH7.00", "TECH10.00", "NIST1.68", "NIST4.01", "NIST6.86", "NIST9.18", "NIST12.68"] ("标液3")
                w317 = u16 5 items=["TECH4.00", "TECH7.00", "TECH10.00", "NIST1.68", "NIST4.01", "NIST6.86", "NIST9.18", "NIST12.68"] ("标液2")
                n166 = local write "三点标液3"(w316) -> ()
                n167 = local write "三点标液2"(w317) -> ()
                n168 = local write "三点标液1"(w315) -> ()
              }
              frame 5..7 {
                w318 = u16 5 items=["TECH4.00", "TECH7.00", "TECH10.00", "NIST1.68", "NIST4.01", "NIST6.86", "NIST9.18", "NIST12.68"] ("标液2")
                w319 = u16 7 items=["TECH4.00", "TECH7.00", "TECH10.00", "NIST1.68", "NIST4.01", "NIST6.86", "NIST9.18", "NIST12.68"] ("标液3")
                w320 = u16 6 items=["TECH4.00", "TECH7.00", "TECH10.00", "NIST1.68", "NIST4.01", "NIST6.86", "NIST9.18", "NIST12.68"] ("标液2")
                n169 = local write "三点标液3"(w319) -> ()
                n170 = local write "三点标液2"(w320) -> ()
                n171 = local write "三点标液1"(w318) -> ()
              }
            }
            n172 = call "Add State to Queue.vi"("State(s) In (\"\")"=w299) -> ("States Out"=w300:string)  [unwired: 14 in]
          }
          event "三点标液2": Value Change {
            n173 = event-data() -> ("NewVal"=w324:u16)  [unwired: 1 in, 5 out]
            n174 = case shown="6, 7" w324 {
              frame 0..2, Default {
                w325 = u16 0 items=["TECH4.00", "TECH7.00", "TECH10.00", "NIST1.68", "NIST4.01", "NIST6.86", "NIST9.18", "NIST12.68"] ("标液2")
                w326 = u16 2 items=["TECH4.00", "TECH7.00", "TECH10.00", "NIST1.68", "NIST4.01", "NIST6.86", "NIST9.18", "NIST12.68"] ("标液3")
                w327 = u16 1 items=["TECH4.00", "TECH7.00", "TECH10.00", "NIST1.68", "NIST4.01", "NIST6.86", "NIST9.18", "NIST12.68"] ("标液2")
                n175 = local write "三点标液3"(w326) -> ()
                n176 = local write "三点标液2"(w327) -> ()
                n177 = local write "三点标液1"(w325) -> ()
              }
              frame 3, 4 {
                w328 = u16 3 items=["TECH4.00", "TECH7.00", "TECH10.00", "NIST1.68", "NIST4.01", "NIST6.86", "NIST9.18", "NIST12.68"] ("标液2")
                w329 = u16 5 items=["TECH4.00", "TECH7.00", "TECH10.00", "NIST1.68", "NIST4.01", "NIST6.86", "NIST9.18", "NIST12.68"] ("标液3")
                w330 = u16 4 items=["TECH4.00", "TECH7.00", "TECH10.00", "NIST1.68", "NIST4.01", "NIST6.86", "NIST9.18", "NIST12.68"] ("标液2")
                n178 = local write "三点标液3"(w329) -> ()
                n179 = local write "三点标液2"(w330) -> ()
                n180 = local write "三点标液1"(w328) -> ()
              }
              frame 5 {
                w331 = u16 6 items=["TECH4.00", "TECH7.00", "TECH10.00", "NIST1.68", "NIST4.01", "NIST6.86", "NIST9.18", "NIST12.68"] ("标液3")
                w332 = u16 5 items=["TECH4.00", "TECH7.00", "TECH10.00", "NIST1.68", "NIST4.01", "NIST6.86", "NIST9.18", "NIST12.68"] ("标液2")
                n181 = local write "三点标液3"(w331) -> ()
                n182 = local write "三点标液2"(w332) -> ()
              }
              frame 6, 7 {
                w333 = u16 7 items=["TECH4.00", "TECH7.00", "TECH10.00", "NIST1.68", "NIST4.01", "NIST6.86", "NIST9.18", "NIST12.68"] ("标液3")
                w334 = u16 6 items=["TECH4.00", "TECH7.00", "TECH10.00", "NIST1.68", "NIST4.01", "NIST6.86", "NIST9.18", "NIST12.68"] ("标液2")
                n183 = local write "三点标液3"(w333) -> ()
                n184 = local write "三点标液2"(w334) -> ()
              }
            }
            n185 = call "Add State to Queue.vi"("State(s) In (\"\")"=w321) -> ("States Out"=w322:string)  [unwired: 14 in]
          }
          event "三点标液3": Value Change {
            n186 = event-data() -> ("NewVal"=w338:u16)  [unwired: 1 in, 5 out]
            n187 = case shown="3..7" w338 {
              frame 0, 1, Default {
                w339 = u16 2 items=["TECH4.00", "TECH7.00", "TECH10.00", "NIST1.68", "NIST4.01", "NIST6.86", "NIST9.18", "NIST12.68"] ("标液2")
                w340 = u16 0 items=["TECH4.00", "TECH7.00", "TECH10.00", "NIST1.68", "NIST4.01", "NIST6.86", "NIST9.18", "NIST12.68"] ("标液3")
                w341 = u16 1 items=["TECH4.00", "TECH7.00", "TECH10.00", "NIST1.68", "NIST4.01", "NIST6.86", "NIST9.18", "NIST12.68"] ("标液2")
                n188 = local write "三点标液3"(w340) -> ()
                n189 = local write "三点标液2"(w341) -> ()
                n190 = local write "三点标液1"(w339) -> ()
              }
              frame 2 {
                w342 = u16 0 items=["TECH4.00", "TECH7.00", "TECH10.00", "NIST1.68", "NIST4.01", "NIST6.86", "NIST9.18", "NIST12.68"] ("标液2")
                w343 = u16 2 items=["TECH4.00", "TECH7.00", "TECH10.00", "NIST1.68", "NIST4.01", "NIST6.86", "NIST9.18", "NIST12.68"] ("标液3")
                w344 = u16 1 items=["TECH4.00", "TECH7.00", "TECH10.00", "NIST1.68", "NIST4.01", "NIST6.86", "NIST9.18", "NIST12.68"] ("标液2")
                n191 = local write "三点标液3"(w343) -> ()
                n192 = local write "三点标液2"(w344) -> ()
                n193 = local write "三点标液1"(w342) -> ()
              }
              frame 3..7 {
                n194 = local read "三点标液1"() -> (w347:u16)
                n195 = local read "三点标液2"() -> (w346:u16)
                n196 = Less?(x=w347, y=w346) -> (x < y?=w345:bool)
                n197 = case shown="假" w345 {
                  frame False {
                  }
                  frame True {
                    n198 = local read "三点标液3"() -> (w350:u16)
                    n199 = local read "三点标液2"() -> (w348:u16)
                    n200 = Less Or Equal?(x=w350, y=w348) -> (x <= y?=w349:bool)
                    n201 = case shown="真" w349 {
                      tunnel: w348 -> [_ w352]
                      frame False {
                      }
                      frame True {
                        n202 = Increment(x=w352) -> (x+1=w351:u16)
                        n203 = local write "三点标液3"(w351) -> ()
                      }
                    }
                  }
                }
              }
            }
            n204 = call "Add State to Queue.vi"("State(s) In (\"\")"=w335) -> ("States Out"=w336:string)  [unwired: 14 in]
          }
          event "标液1", "标液2", "偏移值补偿", "滤波设定": Mouse Down {
            n205 = event-data() -> ("CtlRef"=w359:refnum<vi>)  [unwired: 1 in, 7 out]
            n206 = property class="DigNum (严格)"(reference=w359) -> (reference out=w353:refnum<vi>, "Value"=w354:dbl)  [unwired: 1 in, 1 out]
            n207 = call "数字键盘.vi"("OldNumber"=w354) -> ("NewNumber"=w355:dbl)  [unwired: 1 in]
            n208 = property class="DigNum (严格)"(reference=w353, "Val(Sgnl)"=w355) -> ()  [unwired: 1 in, 2 out]
            n209 = call "Add State to Queue.vi"("State(s) In (\"\")"=w356) -> ("States Out"=w357:string)  [unwired: 14 in]
          }
          event "偏移值补偿": Value Change {
            n210 = event-data() -> ("NewVal"=w364:dbl)  [unwired: 1 in, 5 out]
            n211 = global read "多参数全局变量.vi" "MB session in"() -> (w365:refnum<class "MB_Master.lvclass">)
            n212 = call "000CH_pH_pH偏移修正值写入.vi"("数值"=w364, "MB session in"=w365) -> ("error out"=w362:errorcluster)  [unwired: 8 in, 1 out]
            n213 = Enqueue Element At Opposite End(queue=w363, element=T1."pH" ("元素"), error in (no error)=w362) -> (error out=w361:errorcluster)  [unwired: 1 in, 2 out]
            n214 = call "Add State to Queue.vi"("State(s) In (\"\")"=w368) -> ("States Out"=w367:string)  [unwired: 14 in]
          }
          event "标液1": Value Change {
            n215 = event-data() -> ("NewVal"=w377:dbl)  [unwired: 1 in, 5 out]
            n216 = global read "多参数全局变量.vi" "MB session in"() -> (w375:refnum<class "MB_Master.lvclass">)
            n217 = call "0030H_pH_第一点标准值写入.vi"("数值"=w377, "MB session in"=w375) -> ("error out"=w376:errorcluster)  [unwired: 8 in, 1 out]
            n218 = Enqueue Element At Opposite End(queue=w370, element=T1."pH" ("元素"), error in (no error)=w376) -> (error out=w371:errorcluster)  [unwired: 1 in, 2 out]
            n219 = call "Add State to Queue.vi"("State(s) In (\"\")"=w372) -> ("States Out"=w373:string)  [unwired: 14 in]
          }
          event "标液2": Value Change {
            n220 = event-data() -> ("NewVal"=w386:dbl)  [unwired: 1 in, 5 out]
            n221 = global read "多参数全局变量.vi" "MB session in"() -> (w384:refnum<class "MB_Master.lvclass">)
            n222 = call "0033H_pH_第二点标准值写入.vi"("数值"=w386, "MB session in"=w384) -> ("error out"=w385:errorcluster)  [unwired: 8 in, 1 out]
            n223 = Enqueue Element At Opposite End(queue=w379, element=T1."pH" ("元素"), error in (no error)=w385) -> (error out=w380:errorcluster)  [unwired: 1 in, 2 out]
            n224 = call "Add State to Queue.vi"("State(s) In (\"\")"=w381) -> ("States Out"=w382:string)  [unwired: 14 in]
          }
          event "滤波设定": Value Change {
            n225 = event-data() -> ("NewVal"=w391:dbl)  [unwired: 1 in, 5 out]
            n226 = global read "多参数全局变量.vi" "MB session in"() -> (w392:refnum<class "MB_Master.lvclass">)
            n227 = call "0027H_pH_数位滤波设定写入.vi"("数值"=w391, "MB session in"=w392) -> ("error out"=w390:errorcluster)  [unwired: 8 in, 1 out]
            n228 = Enqueue Element At Opposite End(queue=w388, element=T1."pH" ("元素"), error in (no error)=w390) -> (error out=w389:errorcluster)  [unwired: 1 in, 2 out]
            n229 = call "Add State to Queue.vi"("State(s) In (\"\")"=w393) -> ("States Out"=w394:string)  [unwired: 14 in]
          }
          event "刷新按钮": Value Change {
            n230 = event-data() -> ()  [unwired: 1 in, 6 out]
            n231 = call "Add State to Queue.vi"("State(s) In (\"\")"=w398) -> ("States Out"=w397:string)  [unwired: 14 in]
            n232 = Two Button Dialog(message="请再次确实是否恢复出厂设置！" ("消息")) -> (T button?=w400:bool)  [unwired: 2 in]
            n233 = case shown="真" w400 {
              frame False {
              }
              frame True {
                w401 = u16 33 items=["Factory Reset"=33] ("数值")
                n234 = global read "多参数全局变量.vi" "MB session in"() -> (w402:refnum<class "MB_Master.lvclass">)
                n235 = call "0026H_pH_命令寄存器写入.vi"("数值"=w401, "MB session in"=w402) -> ()  [unwired: 8 in, 2 out]
              }
            }
          }
          event "校准启动": Value Change {
            n236 = event-data() -> ()  [unwired: 1 in, 6 out]
            n237 = global read "多参数全局变量.vi" "校准运行状态"() -> (w404:T6)
            n238 = Bundle By Name(cluster=w404, "ph"=TRUE) -> (w405:T6)
            n239 = call "Add State to Queue.vi"("State(s) In (\"\")"=w409, "State(s) At Back (\"\")"="init: all\nCal: Place standard solution\n Cal: Calibration process\nidle" ("State(s) In (\"\")")) -> ("States Out"=w408:string)  [unwired: 13 in]
            n240 = global write "多参数全局变量.vi" "校准运行状态"(w405) -> ()
          }
          event "校准停止": Value Change {
            n241 = event-data() -> ()  [unwired: 1 in, 6 out]
            n242 = call "Add State to Queue.vi"("State(s) In (\"\")"="init: all\nCal: Over\nidle" ("State(s) In (\"\")")) -> ("States Out"=w411:string)  [unwired: 14 in]
          }
        }
      }
    }
  }
  n243 = while {
    stop <- FALSE stop-if-true
    n244 = global read "多参数全局变量.vi" "权限"() -> (w416:enum16{"一级权限", "二级权限", "三级权限"})
    n245 = Wait (ms)(milliseconds to wait=u32 1000 ("等待时间（毫秒）")) -> ()  [unwired: 1 out]
    n246 = Not Equal?(x=w416, y=enum16{"一级权限", "二级权限", "三级权限"}."一级权限") -> (x != y?=w413:bool)
    n247 = property on="滤波设定" class="DigNum (严格)"("Visible"=w413) -> ()  [unwired: 2 in, 2 out]
    n248 = property on="偏移值补偿" class="DigNum (严格)"("Visible"=w413) -> ()  [unwired: 2 in, 2 out]
  }
